vi "subTiE_Initialize.vi"(11 "Ti Control Lib":refnum<k7>) -> (3 "Ref":T1 caption="TiE Ref (can be hidden)")   [LabVIEW 2015]
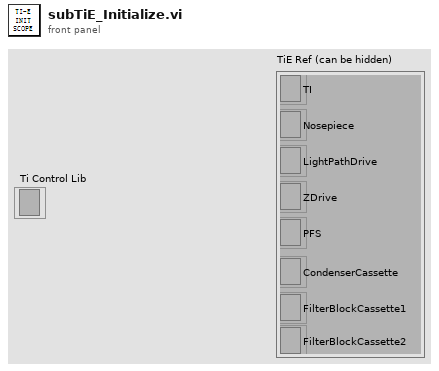
[diagram p1: front panel]
types:
  T1 = cluster{"TI":refnum<k7>, "Nosepiece":refnum<k7>, "LightPathDrive":refnum<k7>, "ZDrive":refnum<k7>, "PFS":refnum<k7>, "CondenserCassette":refnum<k7>, "FilterBlockCassette1":refnum<k7>, "FilterBlockCassette2":refnum<k7>}
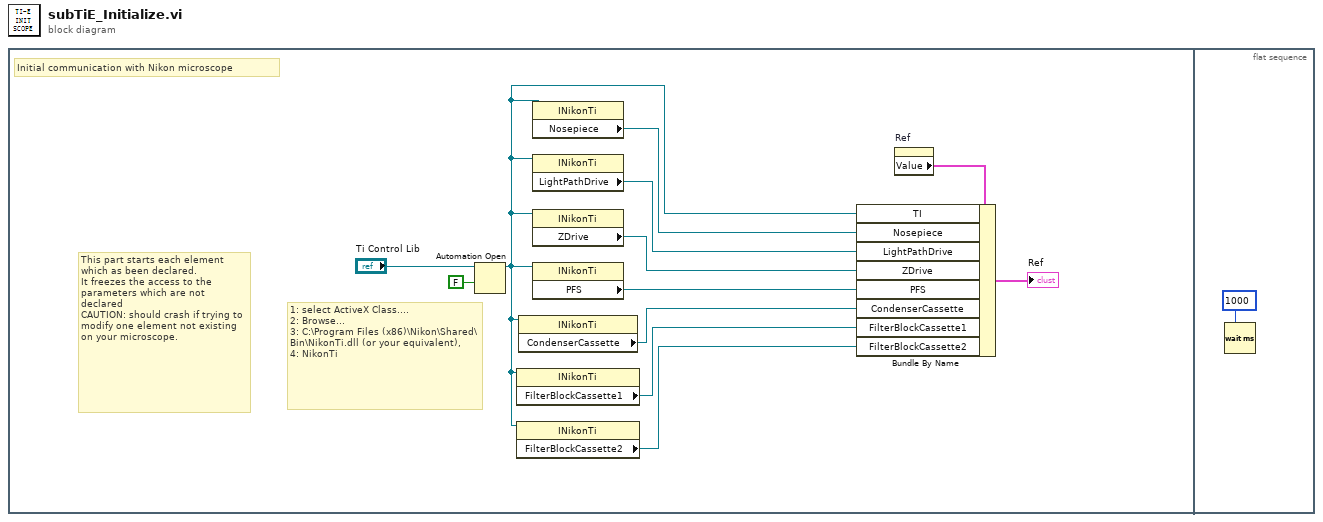
[diagram p0: block diagram]
diagram:
  n1 = flat-sequence {
    frame #0 {
      # "Initial communication with Nikon microscope"
      # "1: select ActiveX Class.... \n2: Browse...\n3: C:\\Program Files (x86)\\Nikon\\Shared\\Bin\\NikonTi.dll (or your equivalent), \n4: NikonTi"
      # "This part starts each element which as been declared. \nIt freezes the access to the parameters which are not declared\nCAUTION: should crash if trying to modify one element not existing on your microscope."
      n2 = Automation Open(Automation Refnum="Ti Control Lib", 9:FALSE ("open new instance (false)")) -> (Automation Refnum=w4:refnum<k7>)  [unwired: 2 in, 1 out]
      n3 = property class="INikonTi"(reference=w4) -> ("FilterBlockCassette1"=w10:refnum<k7>)  [unwired: 1 in, 2 out]
      n4 = property class="INikonTi"(reference=w4) -> ("FilterBlockCassette2"=w11:refnum<k7>)  [unwired: 1 in, 2 out]
      n5 = property class="INikonTi"(reference=w4) -> ("CondenserCassette"=w9:refnum<k7>)  [unwired: 1 in, 2 out]
      n6 = property class="INikonTi"(reference=w4) -> ("Nosepiece"=w5:refnum<k7>)  [unwired: 1 in, 2 out]
      n7 = property class="INikonTi"(reference=w4) -> ("LightPathDrive"=w6:refnum<k7>)  [unwired: 1 in, 2 out]
      n8 = property class="INikonTi"(reference=w4) -> ("ZDrive"=w7:refnum<k7>)  [unwired: 1 in, 2 out]
      n9 = property class="INikonTi"(reference=w4) -> ("PFS"=w8:refnum<k7>)  [unwired: 1 in, 2 out]
      n10 = property on="Ref" class="Clust (strict)"() -> ("Value"=w2:T1)  [unwired: 2 in, 2 out]
      n11 = Bundle By Name(cluster=w2, "TI"=w4, "Nosepiece"=w5, "LightPathDrive"=w6, "ZDrive"=w7, "PFS"=w8, "CondenserCassette"=w9, "FilterBlockCassette1"=w10, "FilterBlockCassette2"=w11) -> (→"Ref":T1)
    }
    frame #1 {
      n12 = Wait (ms)(milliseconds to wait=u32 1000) -> ()  [unwired: 1 out]
    }
  }
